vi "test read UDP.vi"() -> ()   [LabVIEW 2019]
uses:
  Controls/UDP - Command.ctl
  Controls/Communication - Write Data.ctl
  Controls/UDP - Status.ctl
  Controls/UDP - Event.ctl
panel:
  out "Running error":errorcluster
  out "connect error":errorcluster
  out "Channels 2":T1
  out "Data Out":T4 {"Status" items=["Stop", "Ramp Up", "Ramp Down", "Jog Up", "Jog Down", "PID Mode", "PID Ramp"]; "Event" items=["Stop", "Running", "PID", "Up Limit", "Down Limit", "Load Limit"]}
  out "data out":string
  in  "Data":T5={"Test"={"Target Load"=0.0, "Target Disp"=0.0, "Rate"=0.0, "Speed"=0.0}, "Sensor"={"Name"=[], "Unit"=[], "Decimal Point"=[], "Ch Log"=[], "H Alarm"=[], "L Alarm"=[], "H Limit"=[], "L Limit"=[], "Filter"=[], "Gain"=[], "Calib Type"=[]}, "PID"={"SP"=-2.7823365e-08, "PV"=-3.023652e-13, "kP"=8.5432666e-24, "kI"=2.29252e-41, "kD"=1.570387e-38, "FF"=25.0, "Err Band"=0.0, "Max"=15, "Min"=-7, "Ts"=1886611780, "Out"=0, "Mode"=0}, "ADC"={"Active Ch"=[255, 255, 255, 0, 0, 0, 0, 0], "Filter Type"=2, "Post Filter"=[1, 1, 1, 1, 0, 200, 66, 184], "Gain"=[0, 0, 0, 0, 0, 122, 68, 0], "FS"=32, "IntOC"=0, "IntFC"=255, "SysOC"=255, "Cofficient"=[1.0, 1.0, 1.0, 1.0, 1.0, 1.0, 1.0, 1.0], "K"=[1.2450000047683716, 1.2450000047683716], "Max"=1048576}, "System"={"Out Type"=0, "Inverse"=0, "Monitor"=0, "Reserve"=0, "ACC Time"=0, "Pulse Rev"=0, "Stroke"=0, "Auto Off"=0, "Gear Ratio"=0.0, "Pitch"=0.0, "Max Speed"=0, "Jog Speed"=0, "Disp Coff"=0.0, "Max Load"=0}, "Index"=enum."Ch1", "Datalog"=enum."Ch1-Ch16"}
  in  "CMD":T6
  out "Numeric":i32
  in  "stop":bool
  in  "wait":u32
  in  "Array":T7(array[cluster])
  out "Success":bool
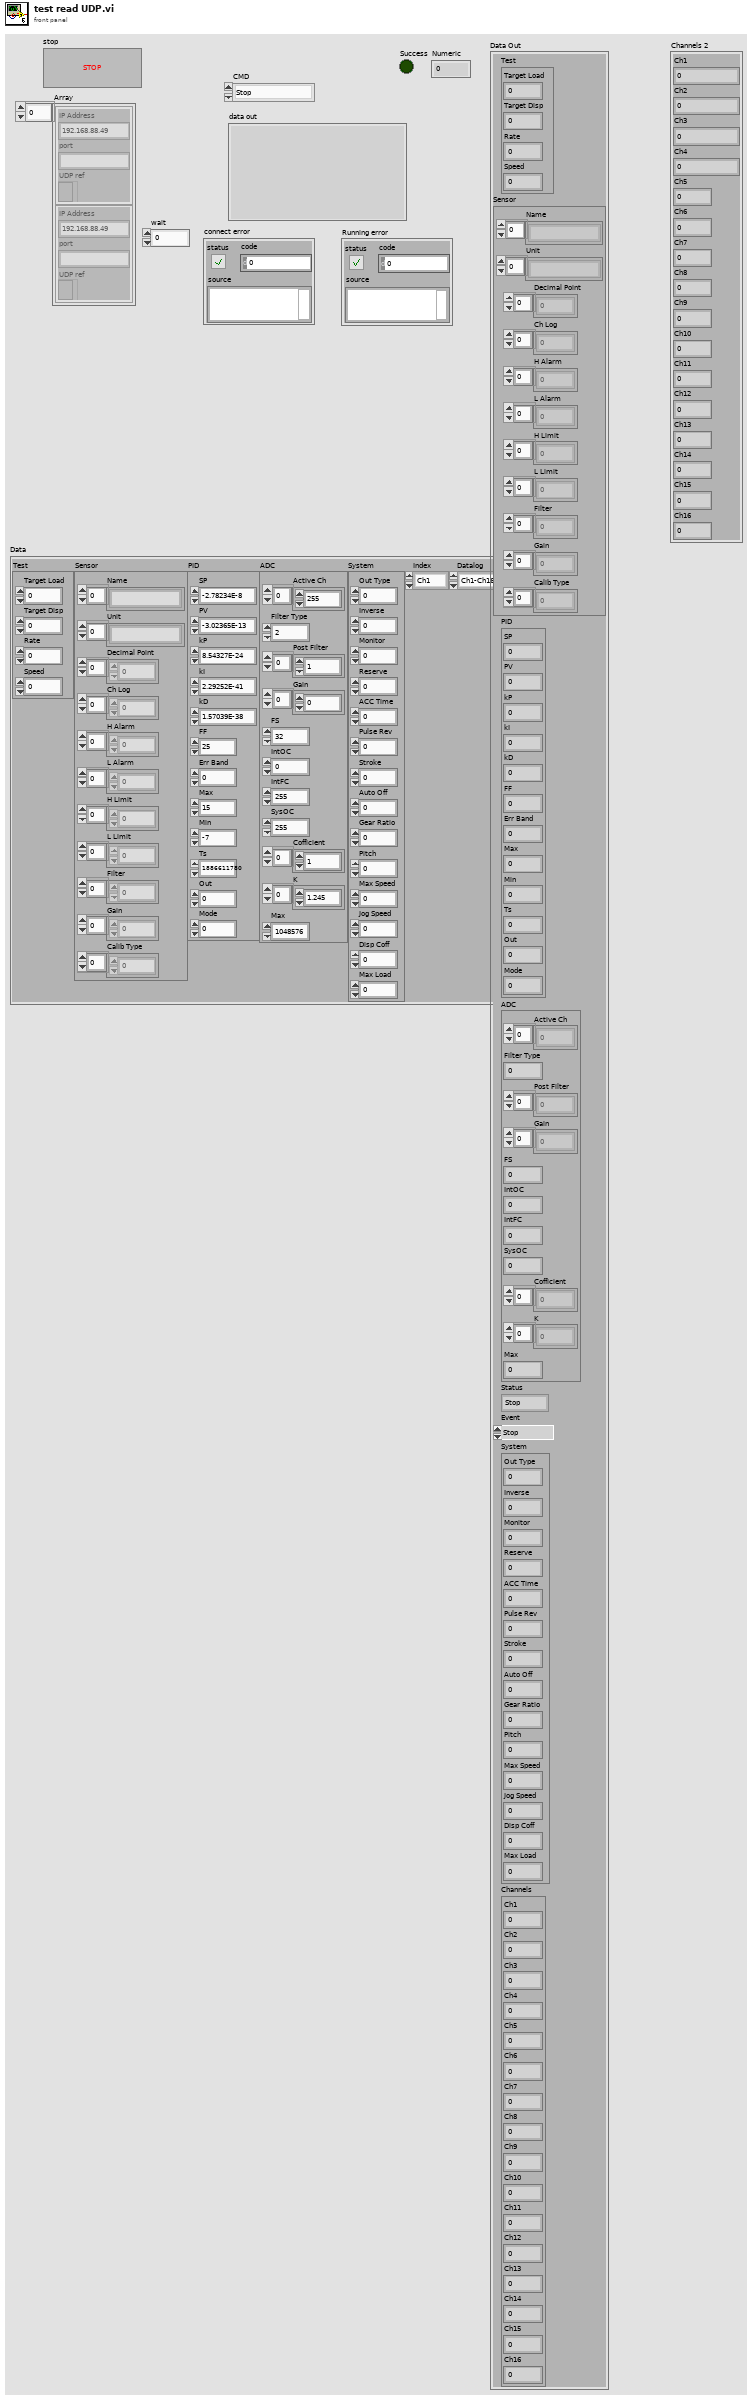
[diagram p1: front panel]
types:
  T1 = cluster{"Ch1":sgl, "Ch2":sgl, "Ch3":sgl, "Ch4":sgl, "Ch5":sgl, "Ch6":sgl, "Ch7":sgl, "Ch8":sgl, "Ch9":sgl, "Ch10":sgl, "Ch11":sgl, "Ch12":sgl, "Ch13":sgl, "Ch14":sgl, "Ch15":sgl, "Ch16":sgl}
  T2 = typedef "UDP - Status.ctl" = u16
  T3 = typedef "UDP - Event.ctl" = u16
  T4 = cluster{"Test":cluster{"Target Load":sgl, "Target Disp":sgl, "Rate":sgl, "Speed":sgl}, "Sensor":cluster{"Name":string[], "Unit":string[], "Decimal Point":u8[], "Ch Log":u8[], "H Alarm":u8[], "L Alarm":u8[], "H Limit":sgl[], "L Limit":sgl[], "Filter":u8[], "Gain":u8[], "Calib Type":u32[]}, "PID":cluster{"SP":sgl, "PV":sgl, "kP":sgl, "kI":sgl, "kD":sgl, "FF":sgl, "Err Band":sgl, "Max":i32, "Min":i32, "Ts":u32, "Out":i32, "Mode":u8}, "ADC":cluster{"Active Ch":u8[], "Filter Type":u8, "Post Filter":u8[], "Gain":u8[], "FS":u16, "IntOC":u8, "IntFC":u8, "SysOC":u8, "Cofficient":dbl[], "K":dbl[], "Max":i32}, "Status":T2, "Event":T3, "System":cluster{"Out Type":u8, "Inverse":u8, "Monitor":u8, "Reserve":u8, "ACC Time":u32, "Pulse Rev":u32, "Stroke":u32, "Auto Off":u32, "Gear Ratio":sgl, "Pitch":sgl, "Max Speed":u32, "Jog Speed":u32, "Disp Coff":sgl, "Max Load":u32}, "Channels":cluster{"Ch1":sgl, "Ch2":sgl, "Ch3":sgl, "Ch4":sgl, "Ch5":sgl, "Ch6":sgl, "Ch7":sgl, "Ch8":sgl, "Ch9":sgl, "Ch10":sgl, "Ch11":sgl, "Ch12":sgl, "Ch13":sgl, "Ch14":sgl, "Ch15":sgl, "Ch16":sgl}}
  T5 = typedef "Communication - Write Data.ctl" = cluster{"Test":cluster{"Target Load":sgl, "Target Disp":sgl, "Rate":sgl, "Speed":sgl}, "Sensor":cluster{"Name":string[], "Unit":string[], "Decimal Point":u8[], "Ch Log":u8[], "H Alarm":u8[], "L Alarm":u8[], "H Limit":sgl[], "L Limit":sgl[], "Filter":u8[], "Gain":u8[], "Calib Type":u32[]}, "PID":cluster{"SP":sgl, "PV":sgl, "kP":sgl, "kI":sgl, "kD":sgl, "FF":sgl, "Err Band":sgl, "Max":i32, "Min":i32, "Ts":u32, "Out":i32, "Mode":u8}, "ADC":cluster{"Active Ch":u8[], "Filter Type":u8, "Post Filter":u8[], "Gain":u8[], "FS":u16, "IntOC":u8, "IntFC":u8, "SysOC":u8, "Cofficient":dbl[], "K":dbl[], "Max":i32}, "System":cluster{"Out Type":u8, "Inverse":u8, "Monitor":u8, "Reserve":u8, "ACC Time":u32, "Pulse Rev":u32, "Stroke":u32, "Auto Off":u32, "Gear Ratio":sgl, "Pitch":sgl, "Max Speed":u32, "Jog Speed":u32, "Disp Coff":sgl, "Max Load":u32}, "Index":enum16{"Ch1", "Ch2", "Ch3", "Ch4", "Ch5", "Ch6", "Ch7", "Ch8", "Ch9", "Ch10", "Ch11", "Ch12", "Ch13", "Ch14", "Ch15", "Ch16"}, "Datalog":enum16{"Ch1-Ch16", "Ch17-Ch32", "Ch32-Ch48", "Ch49-Ch64", "Empty"}}
  T6 = typedef "UDP - Command.ctl" = enum16{"Stop", "Jog Up", "Jog Down", "Ramp Up", "Ramp Down", "PID Target", "PID Ramp", "Disp Run", "Read Ch Data", "Zero Channel", "Zero Disp", "Read Sensor", "Write Sensor", "Read ADC", "Write ADC", "Read PID", "Write PID", "Read Test", "Write Test", "Read System", "Write System", "Read Datalog", "Read Datalog Sensor"}
  T7 = cluster{"IP Address":string, "port":string, "UDP ref":refnum<k16>}[]
  T8 = cluster{"IP Address":string, "port":string, "UDP ref":refnum<k16>}
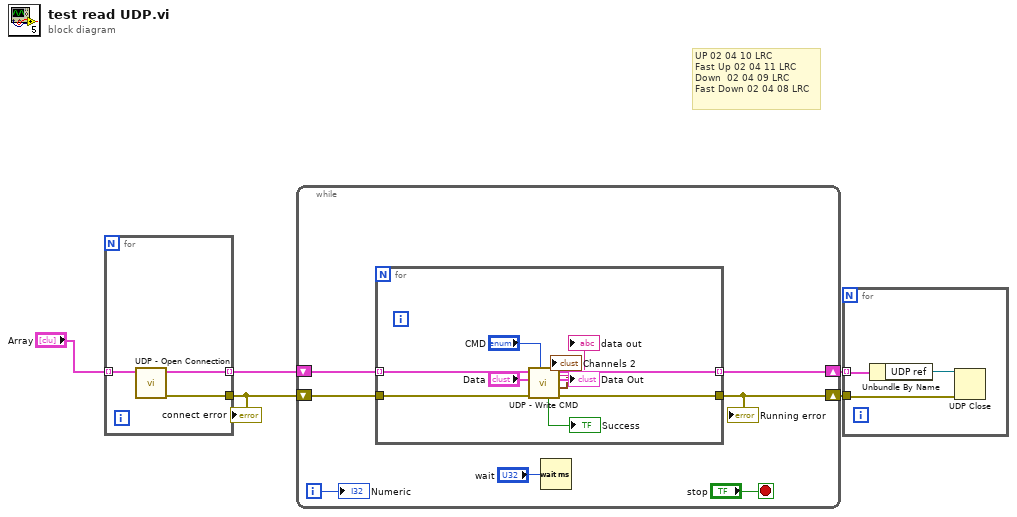
[diagram p0: block diagram]
diagram:
  # "UP 02 04 10 LRC\nFast Up 02 04 11 LRC\nDown  02 04 09 LRC\nFast Down 02 04 08 LRC"
  n1 = for {
    tunnel: [w8] -> w5
    tunnel: [w7] -> w4 mode=indexing
    tunnel: "Array" -> [w6] mode=indexing
    n2 = call "UDP - Open Connection.vi"("UDP Info"=w6) -> ("error out"=w8:errorcluster, "UDP Info Out"=w7:T8)  [unwired: 8 in, 1 out]
  }
  "connect error" <- w5
  n3 = while {
    shift-right: [w13] -> w3
    shift-left: w5 -> [w15]
    shift-right: [w12] -> w2
    shift-left: w4 -> [w14]
    i -> [w10]
    stop <- "stop" stop-if-true
    n4 = for {
      tunnel: w15 -> [w24]
      tunnel: w14 -> [w23] mode=indexing
      tunnel: [w22] -> w13
      tunnel: [w21] -> w12 mode=indexing
      n5 = call "UDP - Write CMD.vi"("CMD"="CMD", "error in"=w24, "Data"="Data", "UDP Info"=w23) -> ("error out"=w22:errorcluster, "Data Out"=→"Data Out":T4, "UDP Info Out"=w21:T8, "Success"=→"Success":bool, "data out"=→"data out":string, "Channels 2"=→"Channels 2":T1)  [unwired: 1 in, 1 out]
    }
    "Running error" <- w13
    n6 = Wait (ms)(milliseconds to wait="wait") -> ()  [unwired: 1 out]
    "Numeric" <- w10
  }
  n7 = for {
    tunnel: w3 -> [w26]
    tunnel: w2 -> [w28] mode=indexing
    n8 = Unbundle By Name(w28) -> ("UDP ref"=w27:refnum<k16>)
    n9 = UDP Close(connection ID=w27, 8:w26) -> ()  [unwired: 2 out]
  }
